vi "File_FilterFiles.vi"(0 "LLB mode":T1(ring), 2 "VIs":T2[](array[typedef]), 4 "Patterns":string[](array[string])) -> (14 "LLB?":bool, 16 "FileNames":string[](array[string]), 17 "FilePaths":path[](array[path]), 18 "TopLevels":bool[](array[boolean]))   [LabVIEW 2010]
uses:
  File_FileInfo.ctl
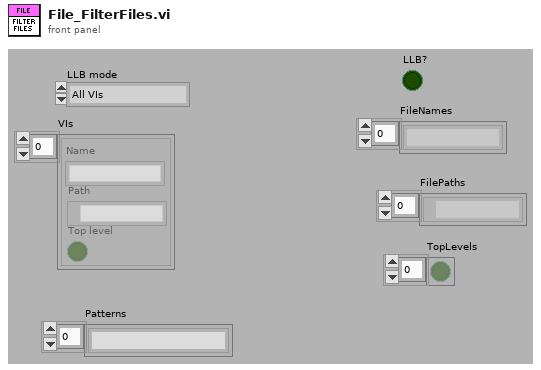
[diagram p1: front panel]
types:
  T1 = enum16{"All VIs", "Only top level", "Only not top level"}
  T2 = typedef "File_FileInfo.ctl" = cluster{"Name":string, "Path":path, "Top level":bool}
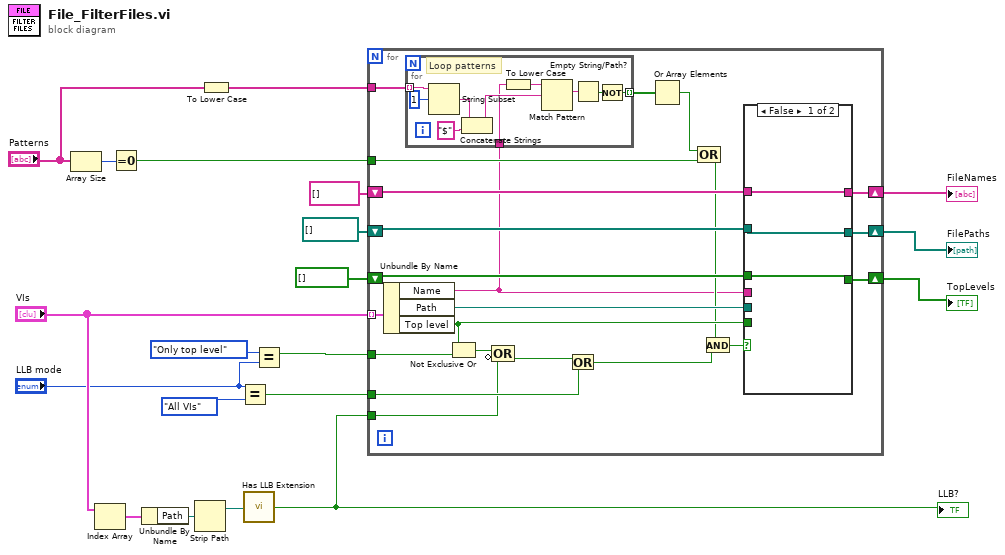
[diagram p0: block diagram]
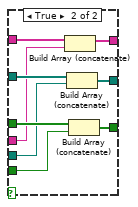
[diagram p2: hidden frame]
diagram:
  n1 = Array Size(array="Patterns") -> (size(s)=w6:i32)
  n2 = Index Array(array="VIs") -> (element=w20:T2)  [unwired: 1 in]
  n3 = Equal To 0?(x=w6) -> (x = 0?=w5:bool)
  n4 = Unbundle By Name(w20) -> ("Path"=w19:path)
  n5 = Strip Path(path=w19) -> (stripped path=w18:path)  [unwired: 1 out]
  n6 = To Lower Case(string="Patterns") -> (all lower case string=w3:string[])
  n7 = Equal?(x="LLB mode", y=T1."All VIs" ("LLB mode")) -> (x = y?=w7:bool)
  n8 = call <vilib>:"Has LLB Extension.vi"("path"=w18) -> ("path to VI library?"=w1:bool)
  "LLB?" <- w1
  n9 = Equal?(x=T1."Only top level" ("LLB mode"), y="LLB mode") -> (x = y?=w2:bool)
  n10 = for {
    tunnel: "VIs" -> [w42] mode=indexing
    shift-right: [w41] -> w13
    shift-left: string[] [] ("FileNames") -> [w40]
    shift-right: [w36] -> w12
    shift-left: path[] [] ("FilePaths") -> [w39]
    shift-right: [w37] -> w11
    shift-left: bool[] [] ("TopLevels") -> [w38]
    tunnel: w7 -> [w34]
    tunnel: w2 -> [w32]
    tunnel: w5 -> [w28]
    tunnel: w3 -> [w27]
    tunnel: w1 -> [w23]
    n11 = Unbundle By Name(w42) -> ("Name"=w26:string, "Path"=w35:path, "Top level"=w33:bool)
    n12 = for {
      tunnel: w27 -> [w52] mode=indexing
      tunnel: w26 -> [w47]
      tunnel: [w44] -> w25 mode=indexing
      # "Loop patterns"
      n13 = String Subset(string=w52, offset (0)=1) -> (substring=w49:string)  [unwired: 1 out]
      n14 = Concatenate Strings(w49, "$") -> (w48:string)
      n15 = To Lower Case(string=w47) -> (all lower case string=w43:string)
      n16 = Match Pattern(string=w43, regular expression=w48) -> (match substring=w46:string)  [unwired: 4 out]
      n17 = Empty String/Path?(string/path=w46) -> (empty?=w45:bool)
      n18 = Not(x=w45) -> (.not. x?=w44:bool)
    }
    n19 = Not Exclusive Or(1:w32, 2:w33) -> (0:w22:bool)
    n20 = Compound Arithmetic op=OR(w22, invert w23) -> (w21:bool)
    n21 = Or(x=w21, y=w34) -> (x .or. y?=w30:bool)
    n22 = Or Array Elements(Boolean array=w25) -> (logical OR=w24:bool)
    n23 = Compound Arithmetic op=OR(w24, w28) -> (w29:bool)
    n24 = And(x=w29, y=w30) -> (x .and. y?=w31:bool)
    n25 = case shown="False" w31 {
      tunnel: [w55 w64] -> w41
      tunnel: w40 -> [w55 w63]
      tunnel: w39 -> [w54 w62]
      tunnel: w38 -> [w53 w61]
      tunnel: [w53 w60] -> w37
      tunnel: [w54 w59] -> w36
      tunnel: w26 -> [_ w58]
      tunnel: w35 -> [_ w57]
      tunnel: w33 -> [_ w56]
      frame False {
      }
      frame True {
        n26 = Build Array (concatenate)(w63, w58) -> (w64:string[])
        n27 = Build Array (concatenate)(w62, w57) -> (w59:path[])
        n28 = Build Array (concatenate)(w61, w56) -> (w60:bool[])
      }
    }
  }
  "FileNames" <- w13
  "FilePaths" <- w12
  "TopLevels" <- w11
